vi "Measure MaxPStabilisation.vi"(4 "Skip pixel?":bool, 6 "Scan settings":T1={"J-V scan"=TRUE, "J-t scan"=FALSE, "Min voltage (V)"=0.0, "Max voltage (V)"=1.4, "Step (V)"=0.01, "Measurement delay (ms)"=10.0, "1st scan FB-SC"=TRUE, "Inverted structure"=FALSE, "Stabilisation time (s)"=0.0, "Stabilisation mode"=0, "Stabilisation value (V or A) "=0.0, "Step time (s)"=1.0, "Integration time"=0, "Repeat light scans"=FALSE, "Stabilisation in the dark?"=FALSE, "J-t Min (V)"=0.0, "J-t Max (V)"=1.4, "J-t Step (V)"=0.01, "Max. power stabilisation"=FALSE, "J-t 1st scan FB-SC"=TRUE, "J-t Inverted structure"=FALSE, "Max power tracking"=FALSE, "Vmp (V)"=0.7, "Total stabilisation time (s)"=100.0, "J-t best pixel only"=0, "Max power best pixel only"=0, "Vmp from J-V scan"=FALSE, "Intensity dependence"=FALSE, "P dep best pixel only"=0, "External quantum efficiency"=FALSE, "EQE best pixel only"=0, "WL min (nm)"=300.0, "WL max (nm)"=900.0, "WL step (nm)"=5.0, "Wait (ms)"=100.0, "No. of repeat scans"=2.0, "Only repeat for best pixel"=0, "Chopper Freq. min (Hz)"=90.0, "Time Constant min (s)"=2.0, "Stabilisation time step (s)"=1.0, "Illumination conditions"=2, "Scan rate min (V/s)"=0.1, "Scan rate max (V/s)"=1.0, "No. of scan rate steps"=1.0, "Scan rate voltage step priority"=FALSE, "Scan rate measurement delay priority"=FALSE, "J-t Illumination conditions"=0, "Chopper Freq. max (Hz)"=200.0, "No. of freq. steps"=1.0, "Time Constant max (s)"=2.0, "No. of t const. steps"=1.0, "White bias min (no. of suns)"=0.1, "White bias max (no. of suns)"=1.0, "No. of white bias steps"=1.0, "Repeat EQE scans"=FALSE, "No. of EQE scans"=2.0, "Max P stab. Specific voltage"=FALSE} {"No. of EQE scans" min=1.0 step=1.0; "No. of white bias steps" min=1.0 step=1.0; "No. of t const. steps" min=1.0 step=1.0; "Time Constant max (s)" items=["0.01s", "0.03s", "0.1s", "0.3s", "1s", "3s"]; "No. of freq. steps" min=1.0 step=1.0; "J-t Illumination conditions" items=["Light only", "Dark only", "Light then dark", "Dark then light"]; "No. of scan rate steps" min=1.0 step=1.0; "Illumination conditions" items=["Light only", "Dark only", "Light then dark", "Dark then light", "Light then dark then light", "Dark then light then dark"]; "Time Constant min (s)" items=["0.01s", "0.03s", "0.1s", "0.3s", "1s", "3s"]; "Only repeat for best pixel" items=["only for best pixel", "for best 2 pixels", "for best 3 pixels", "for best 4 pixels", "for best 5 pixels", "for best 6 pixels", "for best 7 pixels", "for all pixels"]; "No. of repeat scans" min=1.0 step=1.0; "EQE best pixel only" items=["only the best pixel", "the best 2 pixel", "the best 3 pixel", "the best 4 pixel", "the best 5 pixel", "the best 6 pixel", "the best 7 pixel", "all pixels"]; "P dep best pixel only" items=["only the best pixel", "the best 2 pixels", "the best 3 pixels", "the best 4 pixels", "the best 5 pixels", "the best 6 pixels", "the best 7 pixels", "all pixels"]; "Max power best pixel only" items=["only the best pixel", "the best 2 pixels", "the best 3 pixels", "the best 4 pixels", "the best 5 pixels", "the best 6 pixels", "the best 7 pixels", "all pixels"]; "J-t best pixel only" items=["only the best pixel", "the best 2 pixels", "the best 3 pixels", "the best 4 pixels", "the best 5 pixels", "the best 6 pixels", "the best 7 pixels", "all pixels"]; "Integration time" items=["Fast", "Normal", "High Accuracy"]; "Stabilisation mode" items=["V", "I"]; "Measurement delay (ms)" min=10.0}, 7 "Cell details cluster":T3={"Cell Position"=16, "Cell Label"="", "Pixel to measure"=0, "Area (cm^2)"=0.126, "Variable"="", "Variable value"="", "Scan settings in queue"=0, "Light or dark"="", "Measurement Type"=""} {"Pixel to measure" items=["All", "1", "2", "3", "4", "5", "6", "7", "8"]}, 8 "Intensity (no. of suns)":string, 9 "File path of JV log":path, 10 "Experiment Title":string, 11 "User Name":string) -> (3 "Jt Curve":cluster{"Y":dbl[], "Y":dbl[]}[](graph) caption="JV Curve")   [LabVIEW 2011]
uses:
  TypeDefs/Scan settings.ctl
  TypeDefs/Settings Boolean.ctl
  <vilib>/Utility/file.llb/Read From Spreadsheet File (DBL).vi
  <instrlib>/keithley_24xx/Keithley 24XX/Keithley 24XX.lvlib
panel:
  out "File path for Jt image":path
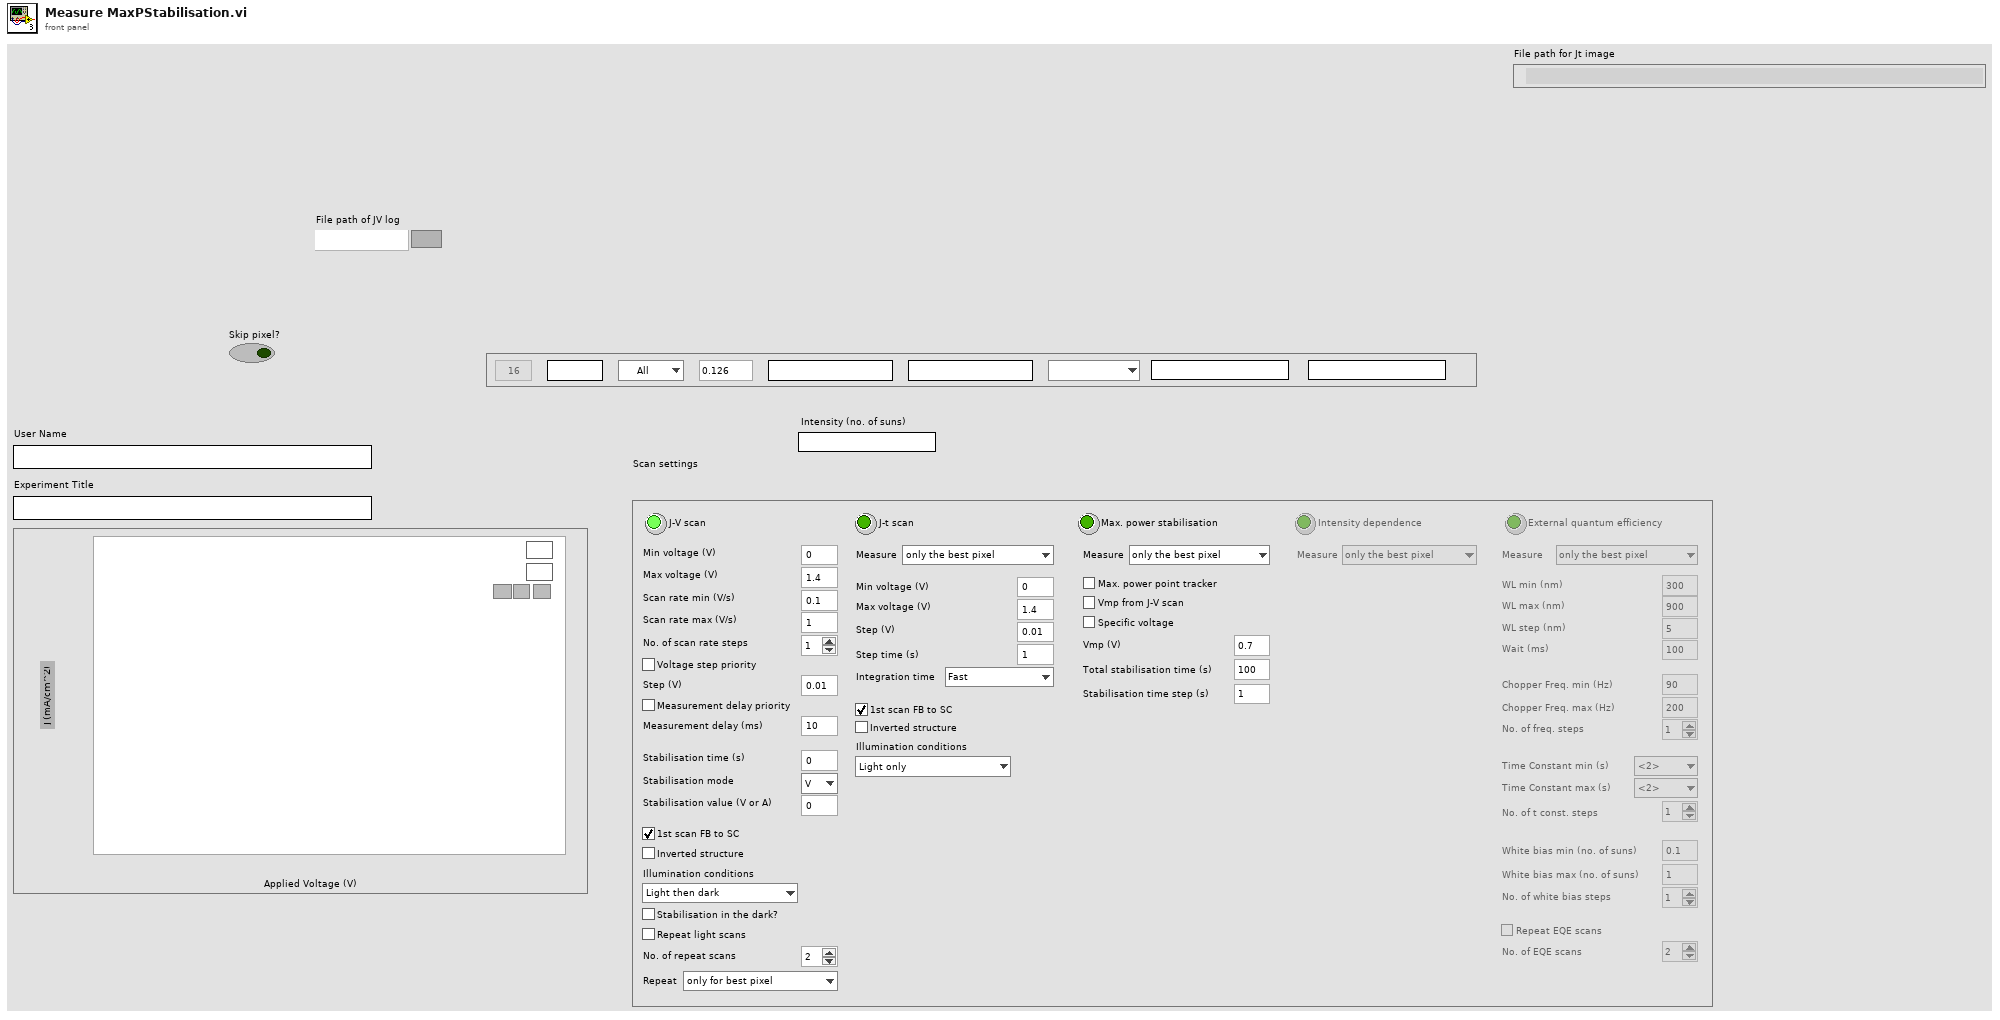
[diagram p1: front panel]
types:
  T1 = typedef "Scan settings.ctl" = cluster{"J-V scan":T2, "J-t scan":bool, "Min voltage (V)":dbl, "Max voltage (V)":dbl, "Step (V)":dbl, "Measurement delay (ms)":dbl, "1st scan FB-SC":bool, "Inverted structure":bool, "Stabilisation time (s)":dbl, "Stabilisation mode":u16, "Stabilisation value (V or A) ":dbl, "Step time (s)":dbl, "Integration time":u16, "Repeat light scans":bool, "Stabilisation in the dark?":bool, "J-t Min (V)":dbl, "J-t Max (V)":dbl, "J-t Step (V)":dbl, "Max. power stabilisation":bool, "J-t 1st scan FB-SC":bool, "J-t Inverted structure":bool, "Max power tracking":bool, "Vmp (V)":dbl, "Total stabilisation time (s)":dbl, "J-t best pixel only":u16, "Max power best pixel only":u16, "Vmp from J-V scan":bool, "Intensity dependence":bool, "P dep best pixel only":u16, "External quantum efficiency":bool, "EQE best pixel only":u16, "WL min (nm)":dbl, "WL max (nm)":dbl, "WL step (nm)":dbl, "Wait (ms)":dbl, "No. of repeat scans":dbl, "Only repeat for best pixel":u16, "Chopper Freq. min (Hz)":dbl, "Time Constant min (s)":dbl, "Stabilisation time step (s)":dbl, "Illumination conditions":u16, "Scan rate min (V/s)":dbl, "Scan rate max (V/s)":dbl, "No. of scan rate steps":dbl, "Scan rate voltage step priority":bool, "Scan rate measurement delay priority":bool, "J-t Illumination conditions":u16, "Chopper Freq. max (Hz)":dbl, "No. of freq. steps":dbl, "Time Constant max (s)":dbl, "No. of t const. steps":dbl, "White bias min (no. of suns)":dbl, "White bias max (no. of suns)":dbl, "No. of white bias steps":dbl, "Repeat EQE scans":bool, "No. of EQE scans":dbl, "Max P stab. Specific voltage":bool}
  T2 = typedef "Settings Boolean.ctl" = bool
  T3 = cluster{"Cell Position":i32, "Cell Label":string, "Pixel to measure":u16, "Area (cm^2)":dbl, "Variable":string, "Variable value":string, "Scan settings in queue":u16, "Light or dark":string, "Measurement Type":string}
  T4 = typedef "imagedata.ctl" = cluster{"image type":i32, "image depth":i32, "image":u8[], "mask":u8[], "colors":u32[], "Rectangle":cluster{"left":i16, "top":i16, "right":i16, "bottom":i16}}
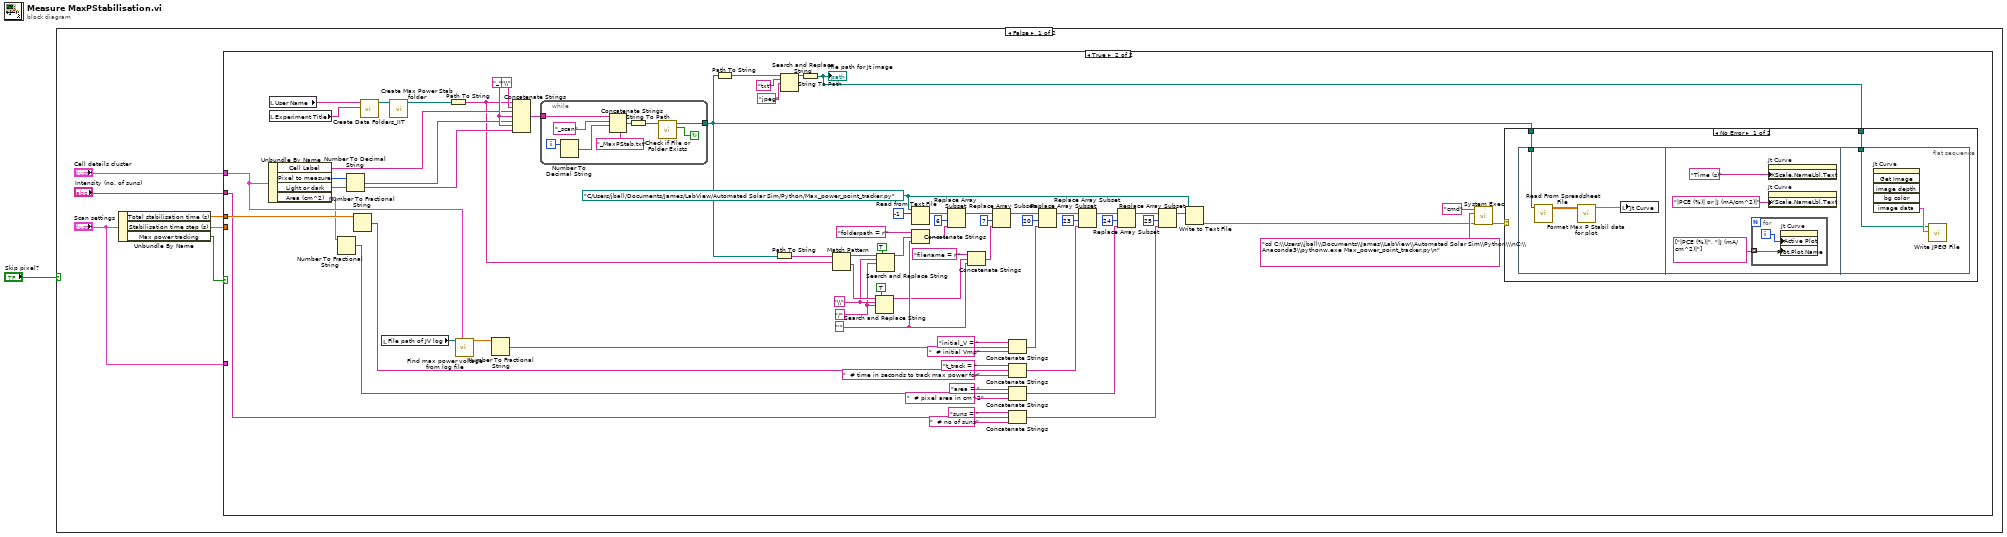
[diagram p0: block diagram]
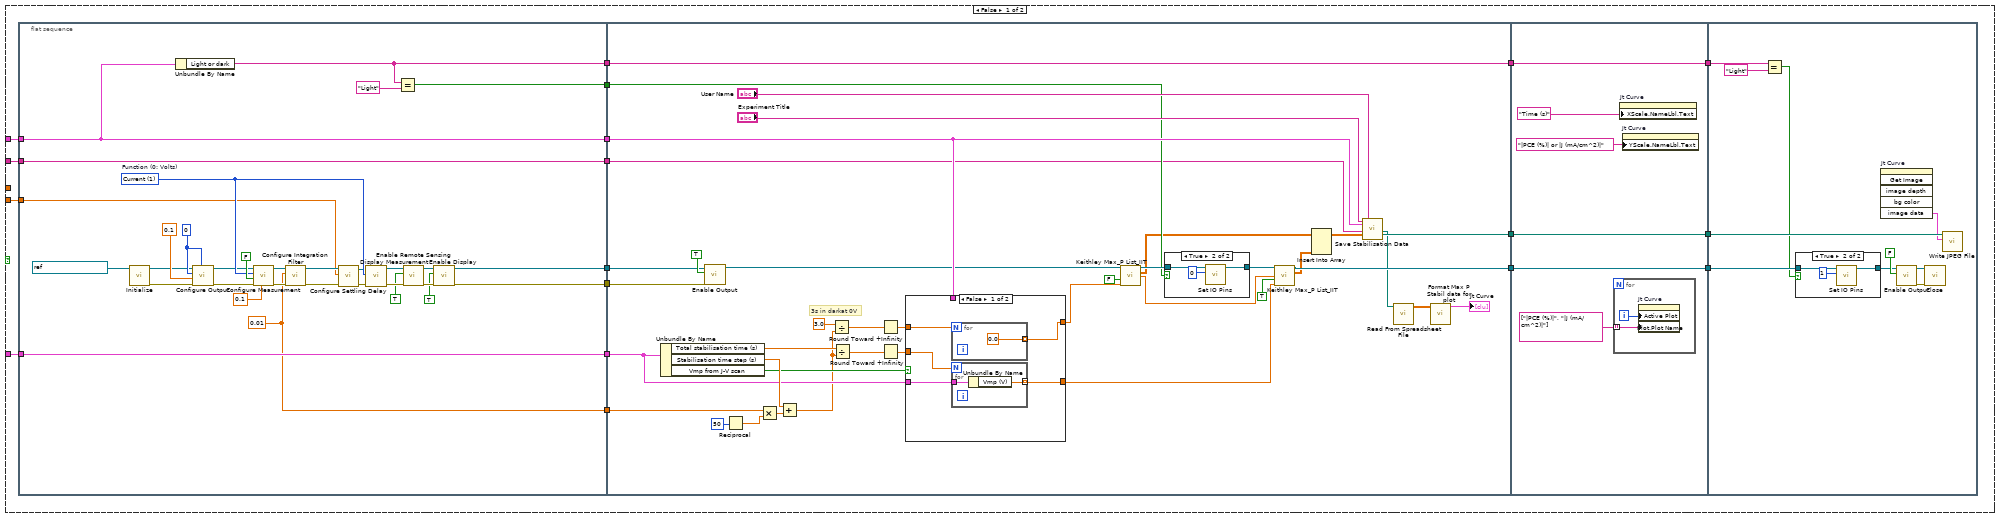
[diagram p2: hidden frame]
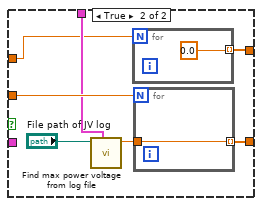
[diagram p4: hidden frame]
diagram:
  n1 = case shown="False" "Skip pixel?" {
    frame False {
      n2 = Unbundle By Name("Scan settings") -> ("Total stabilisation time (s)"=w3:dbl, "Stabilisation time step (s)"=w7:dbl, "Max power tracking"=w4:bool)
      n3 = case shown="True" w4 {
        tunnel: w7 -> [w18 _]
        tunnel: "Cell details cluster" -> [w17 w161]
        tunnel: "Scan settings" -> [w16 _]
        tunnel: w3 -> [_ w168]
        tunnel: "Intensity (no. of suns)" -> [w14 w142]
        frame False {
          n4 = flat-sequence {
            tunnel: [w35] -> w24
            tunnel: [w36] -> w25
            tunnel: [w37] -> w23
            tunnel: w18 -> [w38]
            tunnel: [w40] -> w22
            tunnel: w17 -> [w40]
            tunnel: [w42] -> w21
            tunnel: w16 -> [w42]
            tunnel: [w39] -> w20
            tunnel: [w34] -> w19
            tunnel: [w26] -> w15
            tunnel: w14 -> [w26]
            tunnel: [w94] -> w13
            tunnel: [w96] -> w11
            tunnel: w25 -> [w62]
            tunnel: w24 -> [w61]
            tunnel: w23 -> [w87]
            tunnel: w22 -> [w79]
            tunnel: w21 -> [w82]
            tunnel: [w90] -> w9
            tunnel: w20 -> [w90]
            tunnel: w19 -> [w66]
            tunnel: w15 -> [w60]
            tunnel: w13 -> [w123]
            tunnel: [w123] -> w12
            tunnel: w11 -> [w122]
            tunnel: [w122] -> w10
            tunnel: w9 -> [w121]
            tunnel: [w121] -> w8
            tunnel: w12 -> [w129]
            tunnel: w10 -> [w132]
            tunnel: w8 -> [w126]
            frame #0 {
              w32 = 0
              w37 = 0.01
              w48 = u16 1 items=["Volts", "Current", "Resistance"]  # Function (0: Volts)
              n5 = call <instrlib>:"Initialize.vi"("VISA resource name"=refnum<visa-resource-name> "GPIB0::24::INSTR") -> ("error out"=w27:errorcluster, "VISA resource name out"=w30:refnum<visa-resource-name>)  [unwired: 4 in, 5 out]
              n6 = Unbundle By Name(w40) -> ("Light or dark"=w39:string)
              n7 = call <instrlib>:"Configure Output.vi"("Source Mode  (0: Voltage)"=w32, "error in (no error)"=w27, "Compliance  Level (0.1)"=0.1, "Output Level (0)"=w32, "VISA resource name"=w30) -> ("error out"=w28:errorcluster, "VISA resource name out"=w29:refnum<visa-resource-name>)  [unwired: 5 in]
              n8 = call <instrlib>:"Configure Measurement.vi"("Manual Range (1.0)"=0.1, "error in (no error)"=w28, "Enable Auto Range (T:Enable)"=FALSE, "Function (0: Volts)"=w48, "VISA resource name"=w29) -> ("error out"=w53:errorcluster, "VISA resource name out"=w52:refnum<visa-resource-name>)  [unwired: 5 in]
              n9 = call <instrlib>:"Configure Integration Filter.vi"("error in (no error)"=w53, "Measurement Speed (1 PLC)"=w37, "VISA resource name"=w52) -> ("error out"=w43:errorcluster, "VISA resource name out"=w46:refnum<visa-resource-name>)  [unwired: 7 in]
              n10 = call <instrlib>:"Configure Settling Delay.vi"("error in (no error)"=w43, "Manual Settling Delay (0 sec)"=w38, "VISA resource name"=w46) -> ("error out"=w44:errorcluster, "VISA resource name out"=w45:refnum<visa-resource-name>)  [unwired: 7 in]
              n11 = call <instrlib>:"Display Measurement.vi"("error in (no error)"=w44, "Displayed Measurement (0: Voltage)"=w48, "VISA resource name"=w45) -> ("error out"=w55:errorcluster, "VISA resource name out"=w54:refnum<visa-resource-name>)  [unwired: 7 in]
              n12 = Equal?(x=w39, y="Light") -> (x = y?=w34:bool)
              n13 = call <instrlib>:"Enable Remote Sensing.vi"("error in (no error)"=w55, "Enable Remote Sensing (T: Enable)"=TRUE ("Enable Output (T: Enable)"), "VISA resource name"=w54) -> ("error out"=w50:errorcluster, "VISA resource name out"=w51:refnum<visa-resource-name>)  [unwired: 7 in]
              n14 = call <instrlib>:"Enable Display.vi"("error in (no error)"=w50, "Enable Display (T: Enable)"=TRUE ("Enable Output (T: Enable)"), "VISA resource name"=w51) -> ("error out"=w35:errorcluster, "VISA resource name out"=w36:refnum<visa-resource-name>)  [unwired: 7 in]
            }
            frame #1 {
              # "3s in darkat 0V"
              n15 = Unbundle By Name(w82) -> ("Total stabilisation time (s)"=w84:dbl, "Stabilisation time step (s)"=w85:dbl, "Vmp from J-V scan"=w80:bool)
              n16 = call <instrlib>:"Enable Output.vi"("error in (no error)"=w61, "Enable Output (T: Enable)"=TRUE ("Output (Off)"), "VISA resource name"=w62) -> ("VISA resource name out"=w71:refnum<visa-resource-name>)  [unwired: 7 in, 1 out]
              n17 = Reciprocal(x=50) -> (1/x=w89:dbl)
              n18 = Multiply(x=w87, y=w89) -> (x*y=w86:dbl)
              n19 = Add(x=w85, y=w86) -> (x+y=w78:dbl)
              n20 = Divide(x=3.0, y=w78) -> (x/y=w75:dbl)
              n21 = Divide(x=w84, y=w78) -> (x/y=w76:dbl)
              n22 = Round Toward +Infinity(x=w75) -> (ceil(x): smallest int >= x=w74:dbl)
              n23 = Round Toward +Infinity(x=w76) -> (ceil(x): smallest int >= x=w83:dbl)
              n24 = case shown="False" w80 {
                tunnel: w83 -> [w105 w114]
                tunnel: w82 -> [w103 _]
                tunnel: [w104 w113] -> w81
                tunnel: w79 -> [_ w112]
                tunnel: w74 -> [w102 w111]
                tunnel: [w101 w110] -> w72
                frame False {
                  n25 = for {
                    N: w102 -> [_]
                    tunnel: [0.0 ("Vmp")] -> w101 mode=indexing
                  }
                  n26 = for {
                    N: w105 -> [_]
                    tunnel: w103 -> [w108]
                    tunnel: [w107] -> w104 mode=indexing
                    n27 = Unbundle By Name(w108) -> ("Vmp (V)"=w107:dbl)
                  }
                }
                frame True {
                  n28 = call "Find max power voltage from log file.vi"("Cell details cluster in"=w112, "File path of JV log"="File path of JV log") -> ("Vmp"=w109:dbl)  [unwired: 9 in]
                  n29 = for {
                    N: w111 -> [_]
                    tunnel: [0.0 ("Vmp")] -> w110 mode=indexing
                  }
                  n30 = for {
                    N: w114 -> [_]
                    tunnel: [w117] -> w113 mode=indexing
                    tunnel: w109 -> [w117]
                  }
                }
              }
              n31 = call "Keithley Max_P List_IIT.vi"("VISA resource name in"=w71, "Light?"=FALSE, "Voltage List"=w72) -> ("VISA resource name out"=w68:refnum<visa-resource-name>, "Data Array"=w65:dbl[][], "timestamp"=w67:sgl)  [unwired: 9 in, 1 out]
              n32 = case shown="True" w66 {
                tunnel: w68 -> [w97 w99]
                tunnel: [w97 w98] -> w73
                frame False {
                }
                frame True {
                  n33 = call <instrlib>:"Set IO Pins.vi"("Output Pattern (0)"=0, "VISA resource name"=w99) -> ("VISA resource name out"=w98:refnum<visa-resource-name>)  [unwired: 8 in, 1 out]
                }
              }
              n34 = call "Keithley Max_P List_IIT.vi"("VISA resource name in"=w73, "t=0 timestamp"=w67, "Light?"=TRUE, "Voltage List"=w81) -> ("VISA resource name out"=w94:refnum<visa-resource-name>, "Data Array"=w64:dbl[][])  [unwired: 8 in, 2 out]
              n35 = Insert Into Array(array=w65, new element=w64) -> (w63:dbl[][])  [unwired: 2 in]
              n36 = call "Save Stabilisation Data.vi"("Experiment Indicator"="Experiment Title", "Cell details cluster"=w79, "Intensity (no. of suns)"=w60, "Data Array"=w63, "Username"="User Name") -> ("File path for Jt data"=w59:path, "File path for Jt image"=w96:path)  [unwired: 13 in]
              n37 = call-poly <vilib>:"Read From Spreadsheet File.vi"("file path (dialog if empty)"=w59) -> ("all rows"=w58:dbl[][])  [unwired: 6 in, 4 out]
              n38 = call "Format Max P Stabil data for plot.vi"("Data Array"=w58) -> ("JV Curve"=→"Jt Curve":cluster{"Y":dbl[], "Y":dbl[]}[])  [unwired: 10 in]
            }
            frame #2 {
              n39 = for {
                tunnel: string[] ["|PCE (%)|", "|J (mA/cm^2)|"] ("Measurement queue") -> [w124] mode=indexing
                i -> [w125]
                n40 = property on="Jt Curve" class="XYGraph (strict)"("Active Plot"=w125, "Plot.Plot Name"=w124) -> ()  [unwired: 2 in, 2 out]
              }
              n41 = property on="Jt Curve" class="XYGraph (strict)"("XScale.NameLbl.Text"="Time (s)" ("Y Scale.Name Label.Text")) -> ()  [unwired: 2 in, 2 out]
              n42 = property on="Jt Curve" class="XYGraph (strict)"("YScale.NameLbl.Text"="|PCE (%)| or |J (mA/cm^2)|" ("Y Scale.Name Label.Text")) -> ()  [unwired: 2 in, 2 out]
            }
            frame #3 {
              n43 = Equal?(x=w126, y="Light") -> (x = y?=w127:bool)
              n44 = case shown="True" w127 {
                tunnel: w129 -> [w136 w138]
                tunnel: [w136 w137] -> w128
                frame False {
                }
                frame True {
                  n45 = call <instrlib>:"Set IO Pins.vi"("Output Pattern (0)"=1, "VISA resource name"=w138) -> ("VISA resource name out"=w137:refnum<visa-resource-name>)  [unwired: 8 in, 1 out]
                }
              }
              n46 = invoke on="Jt Curve" class="XYGraph (strict)" method="Get Image"() -> ("image data"=w131:T4)  [unwired: 6 in, 5 out]
              n47 = call <instrlib>:"Enable Output.vi"("Enable Output (T: Enable)"=FALSE ("Output (Off)"), "VISA resource name"=w128) -> ("error out"=w134:errorcluster, "VISA resource name out"=w135:refnum<visa-resource-name>)  [unwired: 8 in]
              n48 = call <instrlib>:"Close.vi"("error in (no error)"=w134, "VISA resource name"=w135) -> ()  [unwired: 9 in, 1 out]
              n49 = call <vilib>:"Write JPEG File.vi"("image data"=w131, "path to JPEG file"=w132) -> ()  [unwired: 8 in, 2 out]
            }
          }
        }
        frame True {
          w175 = "/" ("search string")
          w176 = "\\" ("search string")
          w184 = "'" ("string")
          w186 = path "C:/Users/jball/Documents/James/LabView/Automated Solar Sim/Python/Max_power_point_tracker.py" ("file (use dialog)")
          w203 = "_"
          n50 = Unbundle By Name(w161) -> ("Cell Label"=w199:string, "Pixel to measure"=w200:u16, "Light or dark"=w197:string, "Area (cm^2)"=w151:dbl)
          n51 = local read "User Name"() -> (w206:string)
          n52 = local read "Experiment Title"() -> (w207:string)
          n53 = Number To Fractional String(number=w151) -> (F-format string=w145:string)  [unwired: 3 in]
          n54 = Number To Decimal String(number=w200) -> (decimal integer string=w198:string)  [unwired: 1 in]
          n55 = Number To Fractional String(number=w168) -> (F-format string=w166:string)  [unwired: 3 in]
          n56 = call "Create Data Folders_IIT.vi"("Experiment Indicator"=w207, "username"=w206) -> ("Data Output Folder"=w204:path)  [unwired: 9 in]
          n57 = local read "File path of JV log"() -> (w162:path)
          n58 = call "Create Max Power Stab folder.vi"("Data Folder In"=w204) -> ("Data Output Folder"=w205:path)  [unwired: 10 in]
          n59 = Path To String(path=w205) -> (string=w178:string)
          n60 = call "Find max power voltage from log file.vi"("Cell details cluster in"=w161, "File path of JV log"=w162) -> ("Vmp"=w160:dbl)  [unwired: 9 in]
          n61 = Number To Fractional String(number=w160) -> (F-format string=w157:string)  [unwired: 3 in]
          n62 = Concatenate Strings(w178, "\\", w199, w203, w198, w203, w197) -> (w202:string)
          n63 = while {
            tunnel: w202 -> [w232]
            tunnel: [w224] -> w172
            i -> [w230]
            stop <- w225 continue-if-true
            n64 = Number To Decimal String(number=w230) -> (decimal integer string=w229:string)  [unwired: 1 in]
            n65 = Concatenate Strings(w232, "_scan", w229, "_MaxPStab.txt") -> (w226:string)
            n66 = String To Path(string=w226) -> (path=w227:path)
            n67 = call <vilib>:"Check if File or Folder Exists.vi"("path"=w227) -> ("file or folder exists?"=w225:bool, "dup path"=w224:path)  [unwired: 8 in, 1 out]
          }
          n68 = Path To String(path=w172) -> (string=w211:string)
          n69 = Path To String(path=w172) -> (string=w183:string)
          n70 = Search and Replace String(input string=w211, search string="txt", replace string="jpeg") -> (result string=w208:string)  [unwired: 5 in, 3 out]
          n71 = String To Path(string=w208) -> (path=w170:path)
          "File path for Jt image" <- w170
          n72 = Match Pattern(string=w183, regular expression=w178) -> (before substring=w182:string, after substring=w177:string)  [unwired: 1 in, 2 out]
          n73 = Search and Replace String(replace all?=TRUE ("replace all? (F)"), input string=w177, search string=w176, replace string=w175) -> (result string=w173:string)  [unwired: 4 in, 3 out]
          n74 = Search and Replace String(replace all?=TRUE ("replace all? (F)"), input string=w182, search string=w176, replace string=w175) -> (result string=w181:string)  [unwired: 4 in, 3 out]
          n75 = Read from Text File(file (use dialog)=w186, count=-1) -> (text=w179:string[])  [unwired: 2 in, 3 out]
          n76 = Concatenate Strings("folderpath = r'" ("string"), w181, w184) -> (w190:string)
          n77 = Replace Array Subset(array=w179, new element=w190, index=6) -> (w192:string[])
          n78 = Concatenate Strings("filename = r'" ("string"), w173, w184) -> (w188:string)
          n79 = Replace Array Subset(array=w192, new element=w188, index=7) -> (w155:string[])
          n80 = Concatenate Strings("initial_V = " ("string"), w157, "  # initial Vmp" ("string")) -> (w153:string)
          n81 = Concatenate Strings("t_track = " ("string"), w166, "  # time in seconds to track max power for" ("string")) -> (w152:string)
          n82 = Concatenate Strings("area = " ("string"), w145, "  # pixel area in cm^2" ("string")) -> (w148:string)
          n83 = Concatenate Strings("suns = " ("string"), w142, "  # no of suns" ("string")) -> (w141:string)
          n84 = Replace Array Subset(array=w155, new element=w153, index=20) -> (w154:string[])
          n85 = Replace Array Subset(array=w154, new element=w152, index=23) -> (w169:string[])
          n86 = Replace Array Subset(array=w169, new element=w148, index=24) -> (w146:string[])
          n87 = Replace Array Subset(array=w146, new element=w141, index=25) -> (w140:string[])
          n88 = Write to Text File(file (use dialog)=w186, text=w140) -> (error out=w187:errorcluster)  [unwired: 2 in, 2 out]
          n89 = call <vilib>:"System Exec.vi"("error in (no error)"=w187, "standard input"="cd C:\\Users\\jball\\Documents\\James\\LabView\\Automated Solar Sim\\Python\\\nC:\\Anaconda3\\pythonw.exe Max_power_point_tracker.py\n", "command line"="cmd") -> ("error out"=w171:errorcluster)  [unwired: 5 in, 3 out]
          n90 = case shown="No Error" w171 {
            tunnel: w172 -> [w213 _]
            tunnel: w170 -> [w212 _]
            frame No Error {
              n91 = flat-sequence {
                tunnel: w213 -> [w216]
                tunnel: w212 -> [w222]
                frame #0 {
                  n92 = call-poly <vilib>:"Read From Spreadsheet File.vi"("file path (dialog if empty)"=w216) -> ("all rows"=w215:dbl[][])  [unwired: 6 in, 4 out]
                  n93 = call "Format Max P Stabil data for plot.vi"("Data Array"=w215) -> ("JV Curve"=w214:cluster{"Y":dbl[], "Y":dbl[]}[])  [unwired: 10 in]
                  n94 = local write "Jt Curve"(w214) -> ()
                }
                frame #1 {
                  n95 = for {
                    tunnel: string[] ["|PCE (%)|", "|J (mA/cm^2)|"] ("Measurement queue") -> [w220] mode=indexing
                    i -> [w221]
                    n96 = property on="Jt Curve" class="XYGraph (strict)"("Active Plot"=w221, "Plot.Plot Name"=w220) -> ()  [unwired: 2 in, 2 out]
                  }
                  n97 = property on="Jt Curve" class="XYGraph (strict)"("XScale.NameLbl.Text"="Time (s)" ("Y Scale.Name Label.Text")) -> ()  [unwired: 2 in, 2 out]
                  n98 = property on="Jt Curve" class="XYGraph (strict)"("YScale.NameLbl.Text"="|PCE (%)| or |J (mA/cm^2)|" ("Y Scale.Name Label.Text")) -> ()  [unwired: 2 in, 2 out]
                }
                frame #2 {
                  n99 = invoke on="Jt Curve" class="XYGraph (strict)" method="Get Image"() -> ("image data"=w223:T4)  [unwired: 6 in, 5 out]
                  n100 = call <vilib>:"Write JPEG File.vi"("image data"=w223, "path to JPEG file"=w222) -> ()  [unwired: 8 in, 2 out]
                }
              }
            }
            frame Error {
            }
          }
        }
      }
    }
    frame True {
    }
  }
